vi "Cluster to gRPC LabVIEW Message.vi"(7 "Package Name":string, 8 "error in":errorcluster, 11 "Cluster":variant) -> (0 "error out":errorcluster, 3 "gRPC Message Metadata []":T1[](array[typedef]))   [LabVIEW 2019, in "gprc-lvsupport.lvlib"]
uses:
  gprc-lvsupport.lvlib
  typeDefs/Message Metadata.ctl
  typeDefs/Message Element Metadata.ctl
  typeDefs/Message Element Type.ctl
  <vilib>/Utility/Data Type/NI_Data Type.lvlib
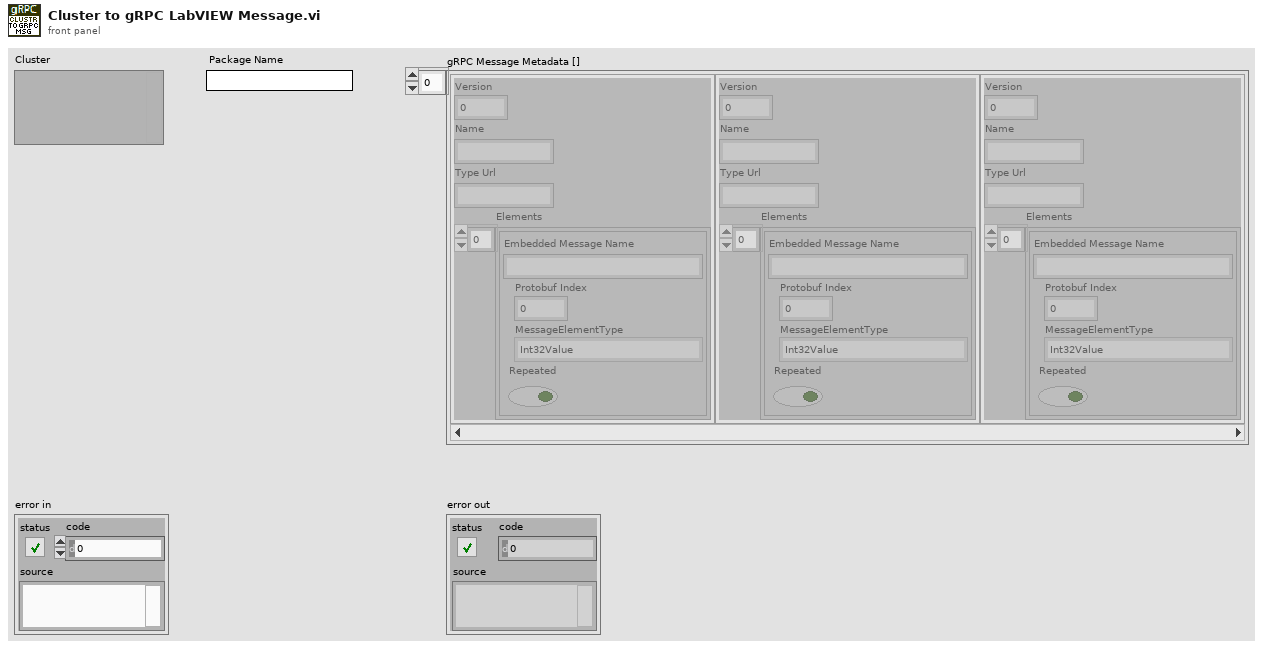
[diagram p1: front panel]
types:
  T1 = typedef "gprc-lvsupport.lvlib/Message Metadata.ctl" = cluster{"Version":i32, "Name":string, "Type Url":string, "Elements":T2[]}
  T2 = typedef "gprc-lvsupport.lvlib/Message Element Metadata.ctl" = cluster{"Embedded Message Name":string, "Protobuf Index":i32, "MessageElementType":T3, "Repeated":bool}
  T3 = typedef "gprc-lvsupport.lvlib/Message Element Type.ctl" = enum32{"Int32Value", "FloatValue", "DoubleValue", "BoolValue", "StringValue", "MessageValue", "Int64Value", "UInt32Value", "UInt64Value", "EnumValue", "Bytes", "Fixed64", "Fixed32", "SFixed64", "SFixed32", "SInt64", "SInt32"}
  T4 = typedef "NI_Data Type.lvlib/Data Type.ctl" = enum8{"Invalid Type", "Void", "I8", "I16", "I32", "I64", "U8", "U16", "U32", "U64", "Single Float", "Double Float", "Extended Float", "Single Complex", "Double Complex", "Extended Complex", "Enum U8", "Enum U16", "Enum U32", "Enum U64", "Single Float With Unit", "Double Float With Unit", "Extended Float With Unit", "Single Complex with Unit", "Double Complex with Unit", "Extended Complex with Unit", "Boolean", "String", "Path", "Picture", "Tag", "Array", "Cluster", "Variant", "LV Variant", "Waveform", "Timestamp", "Digital Waveform", "Digital Data", "ExpressData", "Refnum", "External Data", "VI", "Poly VI", "LabVIEW Class Instance", "Fixed Point", "Set Collection", "Map Collection"}
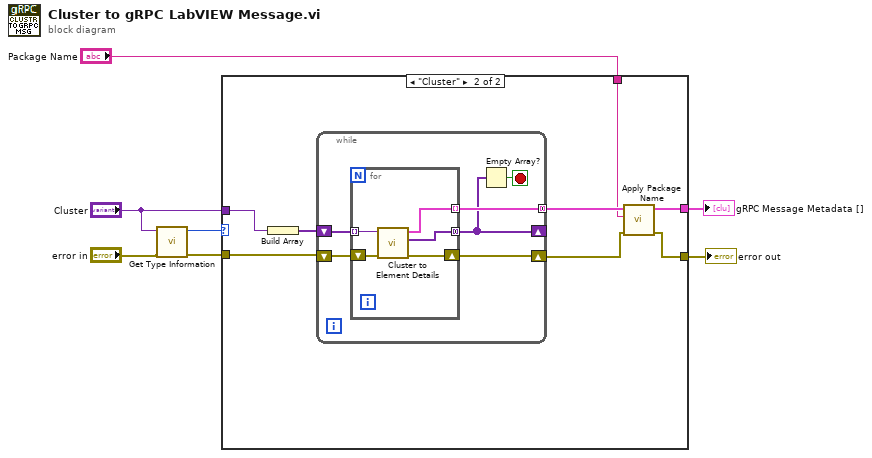
[diagram p0: block diagram]
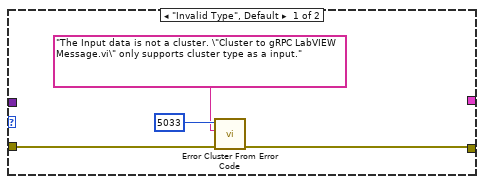
[diagram p2: hidden frame]
diagram:
  n1 = call <vilib>:"Get Type Information.vi"("error in (no error)"="error in", "variant"="Cluster") -> ("error out"=w5:errorcluster, "type"=w2:T4)  [unwired: 5 in, 3 out]
  n2 = case shown="\"Cluster\"" w2 {
    tunnel: [_ w14] -> w4
    tunnel: [w10 w18] -> w7
    tunnel: "Package Name" -> [_ w13]
    tunnel: w5 -> [w11 w17]
    tunnel: "Cluster" -> [_ w12]
    frame "Invalid Type", Default {
      n3 = call <vilib>:"Error Cluster From Error Code.vi"("error in (no error)"=w11, "error message (\"\")"="The Input data is not a cluster. \"Cluster to gRPC LabVIEW Message.vi\" only supports cluster type as a input." ("error message (\"\")"), "error code (0)"=5033) -> ("error out"=w10:errorcluster)  [unwired: 6 in]
    }
    frame "Cluster" {
      n4 = Build Array(w12) -> (w16:variant[])
      n5 = while {
        shift-right: [w20] -> _
        shift-left: w16 -> [w23]
        tunnel: [w22] -> w15 mode=concatenating
        shift-right: [w25] -> w19
        shift-left: w17 -> [w24]
        stop <- w21 stop-if-true
        n6 = for {
          tunnel: [w28] -> w20 mode=concatenating
          tunnel: w23 -> [w27] mode=indexing
          tunnel: [w26] -> w22 mode=indexing
          shift-right: [w30] -> w25
          shift-left: w24 -> [w29]
          n7 = call "Cluster to Element Details.vi"("error in"=w29, "Cluster"=w27) -> ("error out"=w30:errorcluster, "More Cluster"=w28:variant[], "gRPC Message Metadata"=w26:T1)  [unwired: 7 in]
        }
        n8 = Empty Array?(array=w20) -> (empty?=w21:bool)
      }
      n9 = call "Apply Package Name.vi"("error in"=w19, "Package Name"=w13, "gRPC Message Metadata in"=w15) -> ("error out"=w18:errorcluster, "gRPC Message Metadata"=w14:T1[])  [unwired: 7 in]
    }
  }
  "gRPC Message Metadata []" <- w4
  "error out" <- w7
